vi "Memory.Pointer.U64.Write.vi"(8 "error in (no error)":errorcluster, 10 "value":u64, 11 "U64 Pointer in":refnum<class "Memory.Pointer.U64.lvclass">) -> (0 "error out":errorcluster, 2 "value out":u64, 3 "U64 Pointer out":refnum<class "Memory.Pointer.U64.lvclass">)   [LabVIEW 2016, in "LabVIEW Memory Manager.lvlib" / "Memory.Pointer.U64.lvclass"]
uses:
  Memory.Pointer.U64.lvclass
  C:/Users/Ryan/Documents/Git/Sourcetree/LabVIEW-Memory-Manager/Source/Library/Classes/Pointer/Memory.Pointer.lvclass
  Pointer/Memory.Pointer.lvclass/Memory.Pointer.ctl
  Pointer/Memory.Pointer.lvclass
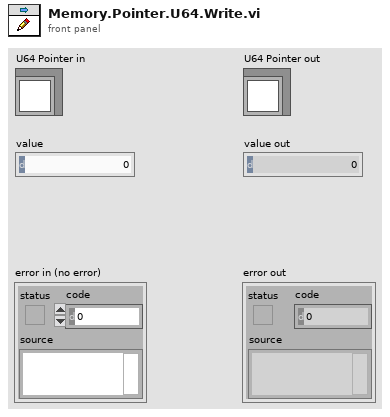
[diagram p1: front panel]
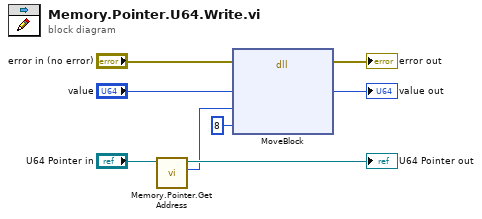
[diagram p0: block diagram]
diagram:
  n1 = call "Memory.Pointer.Get Address.vi"("Pointer in"="U64 Pointer in") -> ("address"=w1:u64, "Pointer out"=→"U64 Pointer out":refnum<class "Memory.Pointer.U64.lvclass">)  [unwired: 8 in, 1 out]
  n2 = dll-call lib="LabVIEW" fn="MoveBlock"(error in="error in (no error)", "src"="value", "dst"=w1, "size"=u64 8) -> (error out=→"error out":errorcluster, "src"=→"value out":u64)  [unwired: 5 in, 1 out]
